vi "layout.vi"(0 "reference":refnum<class "SystemNode.lvclass">, 1 "graph":refnum<class "Graph.lvclass">, 2 "graphics":refnum<class "Graphics.lvclass">, 3 "grid":refnum<class "Grid.lvclass">, 5 "error in (no error)":errorcluster) -> (14 "reference out":refnum<class "SystemNode.lvclass">, 19 "error out":errorcluster)   [LabVIEW 2014, in "SystemNode.lvclass"]
doc: "public void draw(Graphics2D g2)"
uses:
  <resource>/Framework/Providers/Open_GDS/UML/SystemNode_class/SystemNode.lvclass
  <resource>/Framework/Providers/Open_GDS/UML/Grid_class/Grid.lvclass
  <resource>/Framework/Providers/Open_GDS/UML/Graphics_class/Graphics.lvclass
  <resource>/Framework/Providers/Open_GDS/UML/Graph_class/Graph.lvclass
  <resource>/Framework/Providers/Open_GDS/UML/General/Rectangle/Rectangle Rectangle2D.ctl
  <resource>/Framework/Providers/Open_GDS/UML/MultiLineString_class/MultiLineString.lvclass
  <resource>/Framework/Providers/Open_GDS/UML/AbstractNode_class/AbstractNode.lvclass
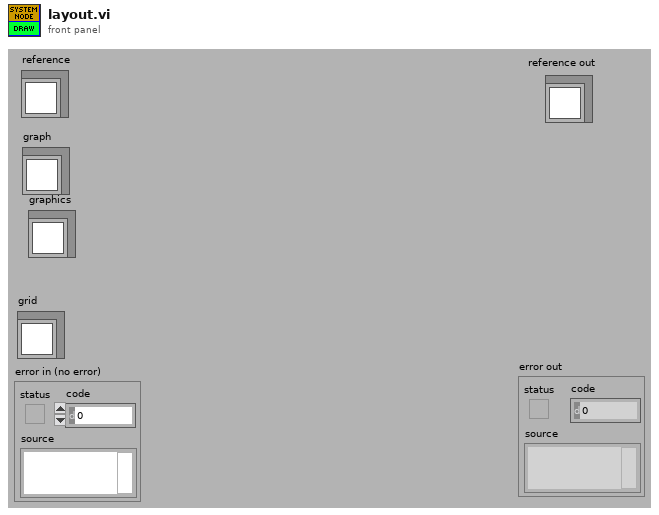
[diagram p1: front panel]
types:
  T1 = typedef "Rectangle Rectangle2D.ctl" = cluster{"x":dbl, "y":dbl, "width":dbl, "height":dbl}
  T2 = typedef "SystemNode.lvclass/ObjectAttributes.ctl" = cluster{"Base class":T3, "contents":refnum<class "MultiLineString.lvclass">, "DEFAULT_WIDTH":i32, "DEFAULT_HEIGHT":i32, "NAME_GAP":i32, "XGAP":i32, "YGAP":i32}
  T3 = typedef "RectangularNode.lvclass/ObjectAttributes.ctl" = cluster{"Base class":T4, "bounds":T1}
  T4 = typedef "AbstractNode.lvclass/ObjectAttributes.ctl" = cluster{"parent":refnum<class "AbstractNode.lvclass">, "children":refnum<class "AbstractNode.lvclass">[], "Hidden":bool}
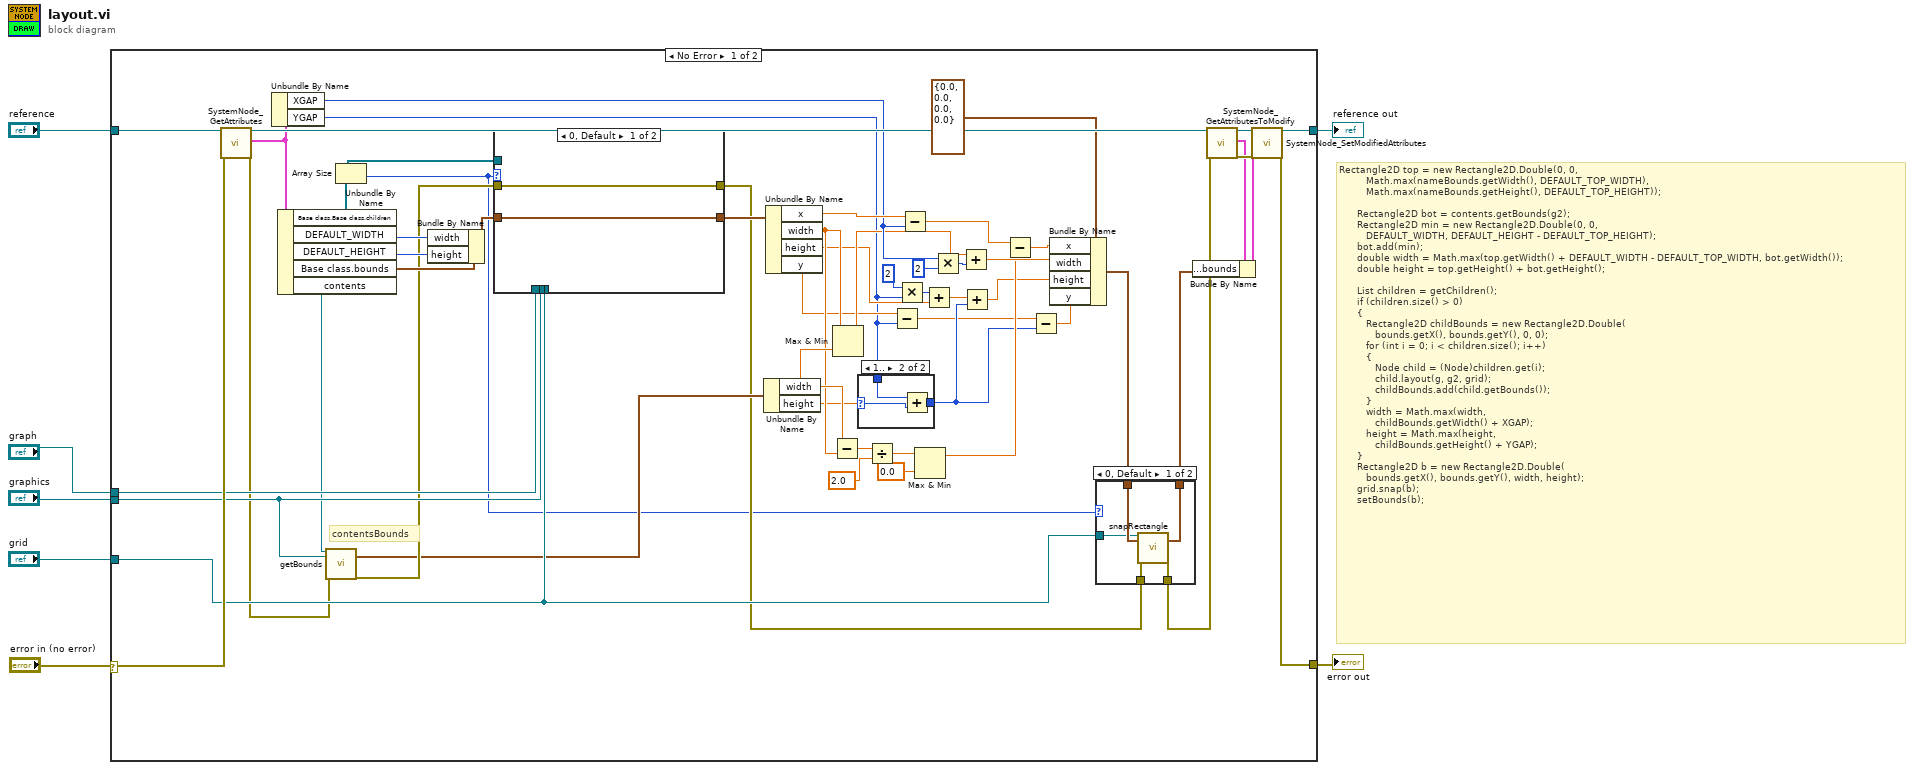
[diagram p0: block diagram]
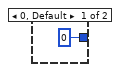
[diagram p3: hidden frame]
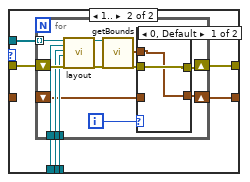
[diagram p4: hidden frame]
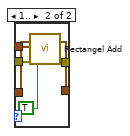
[diagram p5: hidden frame]
diagram:
  # "Rectangle2D top = new Rectangle2D.Double(0, 0,\n         Math.max(nameBounds.getWidth(), DEFAULT_TOP_WIDTH), \n         Math.max(nameBounds.getHeight(), DEFAULT_TOP_HEIGHT));\n\n      Rectangle2D bot = contents.getBounds(g2);\n      Rectangle2D min = new Rectangle2D.Double(0, 0,\n         DEFAULT_WIDTH, DEFAULT_HEIGHT - DEFAULT_TOP_HEIGHT);\n      bot.add(min);\n      double width = Math.max(top.getWidth() + DEFAULT_WIDTH - DEFAULT_TOP_WIDTH, bot.getWidth());\n      double height = top.getHeight() + bot.getHeight();\n\n      List children = getChildren();\n      if (children.size() > 0)\n      {\n         Rectangle2D childBounds = new Rectangle2D.Double(\n            bounds.getX(), bounds.getY(), 0, 0);\n         for (int i = 0; i < children.size(); i++)\n         {\n            Node child = (Node)children.get(i);\n            child.layout(g, g2, grid);\n            childBounds.add(child.getBounds());\n         }\n         width = Math.max(width, \n            childBounds.getWidth() + XGAP);\n         height = Math.max(height, \n            childBounds.getHeight() + YGAP);\n      }\n      Rectangle2D b = new Rectangle2D.Double(\n         bounds.getX(), bounds.getY(), width, height);\n      grid.snap(b);\n      setBounds(b);"
  n1 = case shown="No Error" "error in (no error)" {
    selector: "error in (no error)" -> [w59 w104]
    tunnel: "reference" -> [w62 w105]
    tunnel: [w61 w104] -> w6
    tunnel: [w60 w105] -> w5
    tunnel: "graphics" -> [w58 _]
    tunnel: "grid" -> [w57 _]
    tunnel: "graph" -> [w56 _]
    frame No Error {
      # "contentsBounds"
      n2 = call <resource>:"SystemNode_GetAttributes.vi"("reference in"=w62, "error in (no error)"=w59) -> ("reference out"=w50:refnum<class "SystemNode.lvclass">, "Attributes"=w47:T2, "error out"=w54:errorcluster)  [unwired: 15 out]
      n3 = Unbundle By Name(w47) -> ("XGAP"=w35:i32, "YGAP"=w13:i32)
      n4 = Unbundle By Name(w47) -> ("Base class.Base class.children"=w53:refnum<class "AbstractNode.lvclass">[], "DEFAULT_WIDTH"=w45:i32, "DEFAULT_HEIGHT"=w46:i32, "Base class.bounds"=w44:T1, "contents"=w55:refnum<class "MultiLineString.lvclass">)
      n5 = call-dynamic "getBounds.vi"("reference"=w55, "graphics"=w58, "error in (no error)"=w54) -> ("bounds"=w34:T1, "error out"=w43:errorcluster)  [unwired: 14 in, 1 out]
      n6 = Array Size(array=w53) -> (size(s)=w8:i32)
      n7 = Bundle By Name(cluster=w44, "width"=w45, "height"=w46) -> (w42:T1)
      n8 = case shown="0, Default" w8 {
        tunnel: w43 -> [w75 w82]
        tunnel: w53 -> [_ w81]
        tunnel: w42 -> [w74 _]
        tunnel: [w75 w76] -> w9
        tunnel: w57 -> [_ w80]
        tunnel: w58 -> [_ w79]
        tunnel: w56 -> [_ w78]
        tunnel: [w74 w77] -> w39
        frame 0, Default {
        }
        frame 1.. {
          n9 = for {
            tunnel: w81 -> [w93] mode=indexing
            shift-right: [w95] -> w76
            shift-left: w82 -> [w94]
            shift-right: [w89] -> w77
            shift-left: _ -> [w85]
            tunnel: w80 -> [w88]
            tunnel: w79 -> [w87]
            tunnel: w78 -> [w86]
            i -> [w83]
            n10 = call-dynamic "layout.vi"("reference"=w93, "graph"=w86, "graphics"=w87, "grid"=w88, "error in (no error)"=w94) -> ("reference out"=w92:refnum<class "AbstractNode.lvclass">, "error out"=w91:errorcluster)  [unwired: 13 in]
            n11 = call-dynamic "getBounds.vi"("reference"=w92, "error in (no error)"=w91) -> ("bounds"=w84:T1, "error out"=w90:errorcluster)  [unwired: 15 in, 1 out]
            n12 = case shown="0, Default" w83 {
              tunnel: [w97 w103] -> w95
              tunnel: w90 -> [w97 w102]
              tunnel: [w96 w101] -> w89
              tunnel: w85 -> [_ w100]
              tunnel: w84 -> [w96 w99]
              frame 0, Default {
              }
              frame 1.. {
                n13 = call <resource>:"Rectangel Add.vi"("bounds1"=w100, "bounds2"=w99, "error in (no error)"=w102, "useAbsoluteCordinates(False)"=TRUE) -> ("boundsAdded"=w101:T1, "error out"=w103:errorcluster)  [unwired: 1 in, 13 out]
              }
            }
          }
        }
      }
      n14 = Unbundle By Name(w34) -> ("width"=w32:dbl, "height"=w17:dbl)
      n15 = Unbundle By Name(w39) -> ("x"=w38:dbl, "width"=w31:dbl, "height"=w22:dbl, "y"=w14:dbl)
      n16 = Subtract(x=w32, y=w31) -> (x-y=w28:dbl)
      n17 = Max & Min(x=w31, y=w32) -> (max(x,y)=w33:dbl)  [unwired: 1 out]
      n18 = case shown="1.." w17 {
        selector: w17 -> [_ w73]
        tunnel: w13 -> [_ w72]
        tunnel: [0 w71] -> w16
        frame 0, Default {
        }
        frame 1.. {
          n19 = Add(x=w72, y=w73) -> (x+y=w71:i32)
        }
      }
      n20 = Divide(x=w28, y=2.0) -> (x/y=w26:dbl)
      n21 = Subtract(x=w14, y=w13) -> (x-y=w15:dbl)
      n22 = Multiply(x=2, y=w13) -> (x*y=w21:i32)
      n23 = Subtract(x=w38, y=w35) -> (x-y=w29:dbl)
      n24 = Max & Min(x=w26, y=0.0) -> (max(x,y)=w24:dbl)  [unwired: 1 out]
      n25 = Add(x=w21, y=w22) -> (x+y=w19:dbl)
      n26 = Multiply(x=w35, y=2) -> (x*y=w37:i32)
      n27 = Add(x=w33, y=w37) -> (x+y=w36:dbl)
      n28 = Add(x=w19, y=w16) -> (x+y=w18:dbl)
      n29 = Subtract(x=w29, y=w24) -> (x-y=w30:dbl)
      n30 = Subtract(x=w15, y=w16) -> (x-y=w23:dbl)
      n31 = Bundle By Name(cluster=T1 {"x"=0.0, "y"=0.0, "width"=0.0, "height"=0.0} ("input cluster"), "x"=w30, "width"=w36, "height"=w18, "y"=w23) -> (w12:T1)
      n32 = case shown="0, Default" w8 {
        tunnel: w12 -> [w67 w68]
        tunnel: [w66 w68] -> w11
        tunnel: [w65 w69] -> w10
        tunnel: w9 -> [w64 w69]
        tunnel: w57 -> [w63 _]
        frame 0, Default {
          n33 = call <resource>:"snapRectangle.vi"("reference"=w63, "bounds"=w67, "error in (no error)"=w64) -> ("boundsOut"=w66:T1, "error out"=w65:errorcluster)  [unwired: 15 out]
        }
        frame 1.. {
        }
      }
      n34 = call <resource>:"SystemNode_GetAttributesToModify.vi"("reference in"=w50, "error in (no error)"=w10) -> ("reference out"=w52:refnum<class "SystemNode.lvclass">, "Attributes"=w48:T2, "error out"=w51:errorcluster)  [unwired: 1 in, 14 out]
      n35 = Bundle By Name(cluster=w48, "Base class.bounds"=w11) -> (w49:T2)
      n36 = call <resource>:"SystemNode_SetModifiedAttributes.vi"("reference in"=w52, "Attributes"=w49, "error in (no error)"=w51) -> ("reference out"=w60:refnum<class "SystemNode.lvclass">, "error out"=w61:errorcluster)  [unwired: 3 in, 12 out]
    }
    frame Error {
    }
  }
  "reference out" <- w5
  "error out" <- w6
